vi "lito.vi"() -> ()   [LabVIEW 2016]
panel:
  out "x":dbl
  out "y":dbl
  in  "esp. y2":dbl
  in  "esp. y1":dbl
  in  "esp. x2":dbl
  in  "esp. x1":dbl
  in  "pixel y1":i32
  in  "pixel x1":i32
  in  "ARCHIVO":path
  out "Image":T1(plugin-control)
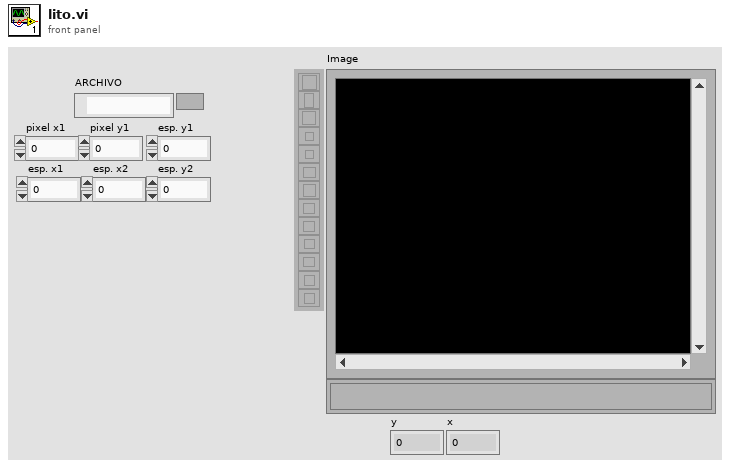
[diagram p1: front panel]
types:
  T1 = typedef "IMAQ Image.ctl" = refnum<image>
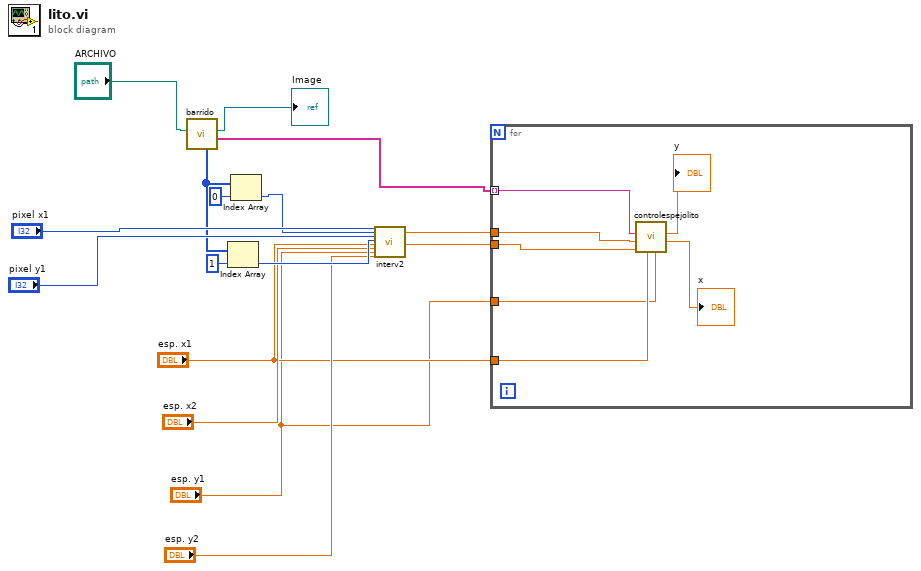
[diagram p0: block diagram]
diagram:
  n1 = call "barrido.vi"("File Path"="ARCHIVO") -> ("ARREGLO DE SALIDA"=w5:string[], "Image"=→"Image":T1, "size(s)"=w12:i32[])  [unwired: 8 in]
  n2 = Index Array(array=w12, index=1) -> (element=w10:i32)
  n3 = Index Array(array=w12, index=0) -> (element=w13:i32)
  n4 = call "interv2.vi"("pixel x1"="pixel x1", "Pixel x2"=w13, "pixel y1"="pixel y1", "pixel y2"=w10, "esp. x1"="esp. x1", "esp. x2"="esp. x2", "esp. y1"="esp. y1", "esp. y2"="esp. y2") -> ("paso x"=w4:dbl, "paso y"=w3:dbl)  [unwired: 18 in]
  n5 = for {
    tunnel: w5 -> [w23] mode=indexing
    tunnel: w4 -> [w22]
    tunnel: w3 -> [w21]
    tunnel: "esp. x1" -> [w20]
    tunnel: "esp. y1" -> [w19]
    n6 = call "controlespejolito.vi"("y inicial"=w19, "x inicial"=w20, "intervalo y"=w21, "intervalo x"=w22, "cadena entrada"=w23) -> ("x"=→"x":dbl, "y"=→"y":dbl)  [unwired: 5 in]
  }
